vi "Stop.vi"(8 "error in (no error)":errorcluster, 10 "Message in":refnum<class "StopMessage.lvclass">, 11 "ExampleClassA in":refnum<class "ExampleClassA.lvclass">) -> (0 "error out":errorcluster, 3 "ExampleClassA out":refnum<class "ExampleClassA.lvclass">)   [LabVIEW 2012, in "ExampleClassA.lvclass"]
doc: "Stops the data production, as well as the streaming to the observer."
uses:
  ExampleClassA.lvclass
  <vilib>/Distrio/Murmex/StopMessage/StopMessage.lvclass
  <vilib>/Distrio/Murmex/Murmex/Murmex.lvclass
  ExampleClassA.lvclass/ExampleClassA.ctl
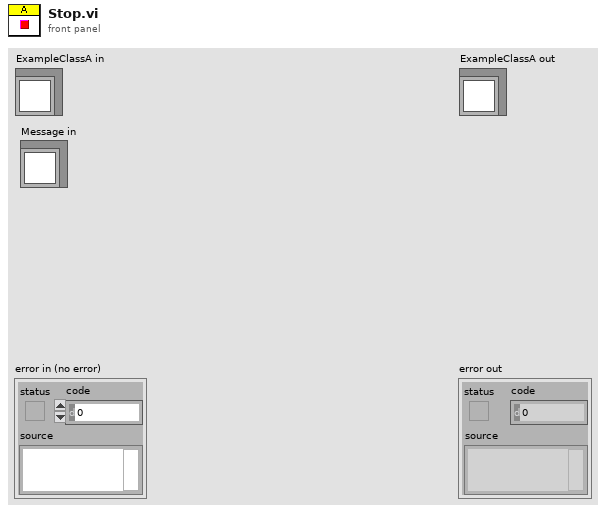
[diagram p1: front panel]
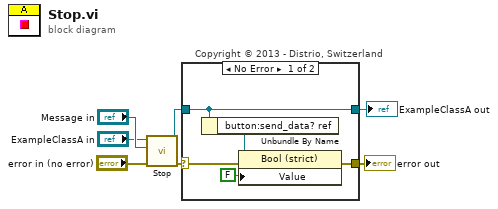
[diagram p0: block diagram]
diagram:
  n1 = call-parent "Stop.vi"("error in (no error)"="error in (no error)", "Message in"="Message in", "Murmex in"="ExampleClassA in") -> ("error out"=w2:errorcluster, "Murmex out"=w4:refnum<class "ExampleClassA.lvclass">)  [unwired: 7 in]
  n2 = case "Copyright © 2013 - Distrio, Switzerland" shown="No Error" w2 {
    selector: w2 -> [w9 w13]
    tunnel: w4 -> [w12 w14]
    tunnel: [w12 w14] -> w3
    tunnel: [w11 w13] -> w1
    frame No Error {
      n3 = Unbundle By Name(w12) -> ("button:send_data? ref"=w10:refnum<vi>)
      n4 = property class="Bool (strict)"(reference=w10, error in=w9, "Value"=FALSE ("Value (Signaling)")) -> (error out=w11:errorcluster)  [unwired: 1 out]
    }
    frame Error {
    }
  }
  "error out" <- w1
  "ExampleClassA out" <- w3
